vi "Remove Child Attributes.vi"(7 "Actor in":refnum<class "Actor.lvclass">, 10 "Alias":string) -> (5 "Actor out":refnum<class "Actor.lvclass">)   [LabVIEW 2020, in "jettl.lvlib"]
uses:
  jettl.lvlib
  Actor/Actor.lvclass
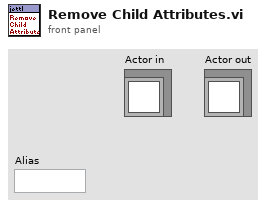
[diagram p1: front panel]
types:
  T1 = typedef "jettl.lvlib/Child Attributes.ctl" = map{string, refnum<data-value>}
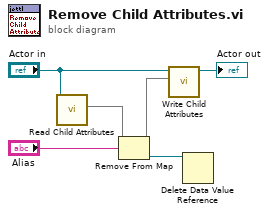
[diagram p0: block diagram]
diagram:
  n1 = call-dynamic "Read Child Attributes.vi"("Actor in"="Actor in") -> ("Child Attributes"=w3:T1)  [unwired: 10 in]
  n2 = Remove From Map(10:"Alias", 11:w3) -> (1:w1:refnum<data-value>, 3:w4:T1)  [unwired: 1 out]
  n3 = call-dynamic "Write Child Attributes.vi"("Child Attributes"=w4, "Actor in"="Actor in") -> ("Actor out"=→"Actor out":refnum<class "Actor.lvclass">)  [unwired: 9 in]
  n4 = Delete Data Value Reference(data value reference=w1) -> ()  [unwired: 1 in, 2 out]
